vi "Excel Easy Graph.vi"(0 "report in":refnum<class "NI_report.lvclass">, 1 "graph title (\"\")":string, 2 "worksheet (\"\")":string, 5 "graph type (col clustered)":i32(ring)=51 items=["xlColumnClustered"=51, "xlColumnStacked"=52, "xlColumnStacked100"=53, "xl3DColumnClustered"=54, "xl3DColumnStacked"=55, "xl3DColumnStacked100"=56, "xlBarClustered"=57, "xlBarStacked"=58, "xlBarStacked100"=59, "xl3DBarClustered"=60, "xl3DBarStacked"=61, "xl3DBarStacked100"=62, "xlLineStacked"=63, "xlLineStacked100"=64, "xlLineMarkers"=65, "xlLineMarkersStacked"=66, "xlLineMarkersStacked100"=67, "xlPieOfPie"=68, "xlPieExploded"=69, "xl3DPieExploded"=70, "xlBarOfPie"=71, "xlXYScatterSmooth"=72, "xlXYScatterSmoothNoMarkers"=73, "xlXYScatterLines"=74, "xlXYScatterLinesNoMarkers"=75, "xlAreaStacked"=76, "xlAreaStacked100"=77, "xl3DAreaStacked"=78, "xl3DAreaStacked100"=79, "xlDoughnutExploded"=80, "xlRadarMarkers"=81, "xlRadarFilled"=82, "xlSurface"=83, "xlSurfaceWireframe"=84, "xlSurfaceTopView"=85, "xlSurfaceTopViewWireframe"=86, "xlBubble"=15, "xlBubble3DEffect"=87, "xlStockHLC"=88, "xlStockOHLC"=89, "xlStockVHLC"=90, "xlStockVOHLC"=91, "xlCylinderColClustered"=92, "xlCylinderColStacked"=93, "xlCylinderColStacked100"=94, "xlCylinderBarClustered"=95, "xlCylinderBarStacked"=96, "xlCylinderBarStacked100"=97, "xlCylinderCol"=98, "xlConeColClustered"=99, "xlConeColStacked"=100, "xlConeColStacked100"=101, "xlConeBarClustered"=102, "xlConeBarStacked"=103, "xlConeBarStacked100"=104, "xlConeCol"=105, "xlPyramidColClustered"=106, "xlPyramidColStacked"=107, "xlPyramidColStacked100"=108, "xlPyramidBarClustered"=109, "xlPyramidBarStacked"=110, "xlPyramidBarStacked100"=111, "xlPyramidCol"=112, "xl3DColumn"=-4100, "xlLine"=4, "xl3DLine"=-4101, "xl3DPie"=-4102, "xlPie"=5, "xlXYScatter"=-4169, "xl3DArea"=-4098, "xlArea"=1, "xlDoughnut"=-4120, "xlRadar"=-4151], 7 "start (0, 0)":cluster{"row":i32, "column":i32}, 9 "data":dbl[][](array[numeric]) format="%.2f", 11 "error in (no error)":errorcluster, 12 "name (\"\")":string, 13 "row headers":string[](array[string]), 14 "column headers":string[](array[string])) -> (4 "report out":refnum<class "NI_report.lvclass">, 15 "error out":errorcluster)   [LabVIEW 2010, in "NI_ReportGenerationToolkit.lvlib"]
doc: "Inserts a graph into a Microsoft Excel report."
uses:
  <vilib>/addons/_office/NI_ReportGenerationToolkit.lvlib
  <vilib>/Utility/NIReport.llb/NI_report.lvclass
  <vilib>/Utility/NIReport.llb/Excel/NI_Excel.lvclass
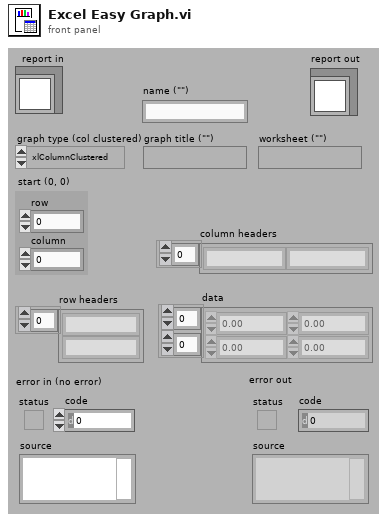
[diagram p1: front panel]
types:
  T1 = cluster{"row":i32, "column":i32, "Height":i32, "Width":i32}
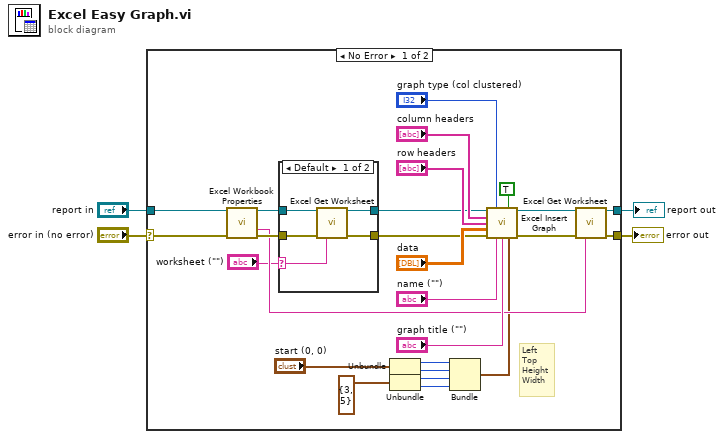
[diagram p0: block diagram]
diagram:
  n1 = case shown="No Error" "error in (no error)" {
    selector: "error in (no error)" -> [w5 w39]
    tunnel: "report in" -> [w20 w38]
    tunnel: [w16 w39] -> w3
    tunnel: [w15 w38] -> w2
    frame No Error {
      # "Left\nTop\nHeight\nWidth"
      n2 = call <vilib>:"Excel Workbook Properties.vi"("report in"=w20, "error in (no error)"=w5) -> ("report out"=w19:refnum<class "NI_report.lvclass">, "current worksheet name"=w14:string, "error out"=w21:errorcluster)  [unwired: 4 in, 7 out]
      n3 = case shown="Default" "worksheet (\"\")" {
        selector: "worksheet (\"\")" -> [w31 _]
        tunnel: [w35 w36] -> w23
        tunnel: [w34 w37] -> w22
        tunnel: w21 -> [w33 w36]
        tunnel: w19 -> [w32 w37]
        frame Default {
          n4 = call <vilib>:"Excel Get Worksheet.vi"("report in"=w32, "error in (no error)"=w33, "name (\"\")"=w31) -> ("report out"=w34:refnum<class "NI_report.lvclass">, "error out"=w35:errorcluster)  [unwired: 1 in, 10 out]
        }
        frame "" {
        }
      }
      n5 = Unbundle("start (0, 0)") -> ("row"=w7:i32, "column"=w8:i32)
      n6 = Unbundle(cluster{"Height":i32, "Width":i32} {"Height"=3, "Width"=5} ("chart size")) -> ("Height"=w11:i32, "Width"=w10:i32)
      n7 = Bundle("row"=w7, "column"=w8, "Height"=w11, "Width"=w10) -> (w9:T1)  [unwired: 1 out]
      n8 = call <vilib>:"Excel Insert Graph.vi"("report in"=w22, "graph type (col clustered)"="graph type (col clustered)", "has legend? (F)"=TRUE ("has legend?"), "column headers"="column headers", "row headers"="row headers", "data"="data", "error in (no error)"=w23, "name (\"\")"="name (\"\")", "graph title (\"\")"="graph title (\"\")", "position/size"=w9) -> ("report out"=w17:refnum<class "NI_report.lvclass">, "error out"=w18:errorcluster)  [unwired: 1 in, 3 out]
      n9 = call <vilib>:"Excel Get Worksheet.vi"("report in"=w17, "error in (no error)"=w18, "name (\"\")"=w14) -> ("report out"=w15:refnum<class "NI_report.lvclass">, "error out"=w16:errorcluster)  [unwired: 1 in, 10 out]
    }
    frame Error {
    }
  }
  "error out" <- w3
  "report out" <- w2
